vi "Ramp Down (2D).vi"(3 "Up (F)":bool, 4 "Array":dbl[][](array[numeric])) -> (1 "Ramped array":dbl[][](array[numeric]))   [LabVIEW 2020]
uses:
  PXI DAQ VIs/Utility VIs/Array Dimensions (2D).vi
  <vilib>/Analysis/NI_AALBase.lvlib
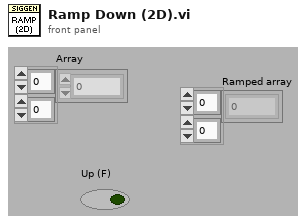
[diagram p1: front panel]
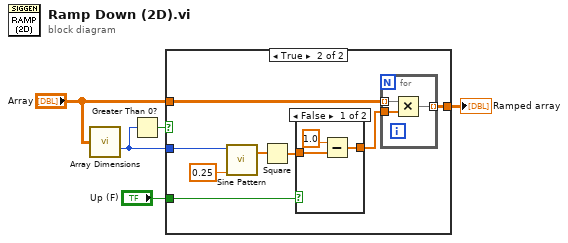
[diagram p0: block diagram]
diagram:
  n1 = call-poly "Array Dimensions.vi"("2D Array"="Array") -> ("# columns"=w2:i32)  [unwired: 13 in, 1 out]
  n2 = Greater Than 0?(x=w2) -> (x > 0?=w5:bool)
  n3 = case shown="True" w5 {
    tunnel: w2 -> [_ w9]
    tunnel: "Array" -> [w6 w12]
    tunnel: [w6 w11] -> w3
    tunnel: "Up (F)" -> [_ w7]
    frame False {
    }
    frame True {
      n4 = call <vilib>:"Sine Pattern.vi"("cycles"=0.25, "samples"=w9) -> ("Sinusoidal Pattern"=w13:dbl[])  [unwired: 2 in, 1 out]
      n5 = Square(x=w13) -> (x^2=w8:dbl[])
      n6 = case shown="False" w7 {
        tunnel: [w17 w18] -> w10
        tunnel: w8 -> [w16 w18]
        frame False {
          n7 = Subtract(x=1.0, y=w16) -> (x-y=w17:dbl[])
        }
        frame True {
        }
      }
      n8 = for {
        tunnel: w12 -> [w21] mode=indexing
        tunnel: w10 -> [w20]
        tunnel: [w19] -> w11 mode=indexing
        n9 = Multiply(x=w21, y=w20) -> (x*y=w19:dbl[])
      }
    }
  }
  "Ramped array" <- w3
